vi "Check Adapter.vi"(8 "error in (no error)":errorcluster, 11 "Authentication Service in":refnum<class "Authentication Service.lvclass">) -> (0 "error out":errorcluster, 3 "Adapter Loaded":bool)   [LabVIEW 2026, in "Authentication Service.lvclass"]
doc: "Checks that the loaded adapter is non-default."
uses:
  Authentication Service.lvclass
  Authentication Service.lvclass/Authentication Service.ctl
  Interfaces/I Authentication Provider/I Authentication Provider.lvclass
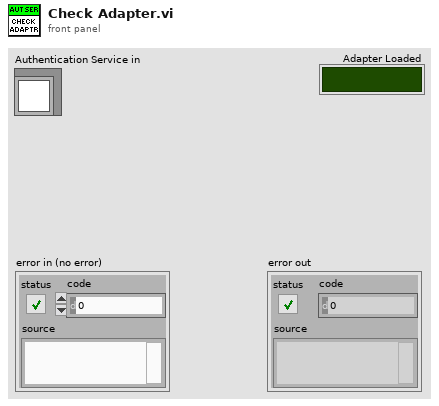
[diagram p1: front panel]
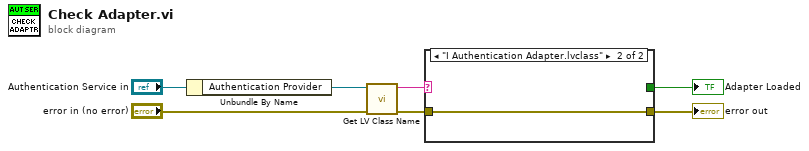
[diagram p0: block diagram]
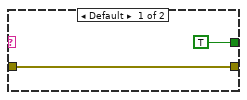
[diagram p2: hidden frame]
diagram:
  n1 = Unbundle By Name("Authentication Service in") -> ("Authentication Provider"=w3:refnum<class "I Authentication Provider.lvclass">)
  n2 = call <vilib>:"Get LV Class Name.vi"("error in (no error)"="error in (no error)", "object"=w3) -> ("error out"=w2:errorcluster, "class name"=w1:string)  [unwired: 8 in]
  n3 = case shown="\"I Authentication Adapter.lvclass\"" w1 {
    tunnel: w2 -> [w8 w10]
    tunnel: [w8 w10] -> w6
    tunnel: [TRUE _] -> w7
    frame Default {
    }
    frame "I Authentication Adapter.lvclass" {
    }
  }
  "Adapter Loaded" <- w7
  "error out" <- w6
